vi "LinearFitAnalysis.vi"() -> ()   [LabVIEW 2014]
uses:
  <vilib>/Analysis/NI_AALBase.lvlib
panel:
  out "XY Graph 2":T1(graph)={"X Values"=[-40.353522941082986, -31.05581354762909, -21.758104154175193, -12.460394760721293, -3.162685367267396, 6.135024026186502, 15.4327334196404, 24.730442813094296, 34.02815220654819, 43.32586160000209], "Histogram: h(x)"=[5, 8, 4, 4, 5, 3, 6, 5, 6, 4]}
  out "Histogram":dynamicdata(graph)=[{"t0"=timestamp(-38.357142857142854 s since 1904-01-01), "dt"=13.285714285714286, "Y"=[7.0, 8.0, 5.0, 8.0, 6.0, 8.0, 7.0], "attributes"=variant("NI_ChannelName"=variant(string "Residual (Histogram)"), "NI_ExpIsRelativeTime"=variant(bool TRUE), "NI_ExpStartTimeStamp"=variant(timestamp timestamp(3625242129.7911425 s since 1904-01-01)), "NI_ExpTimeStamp"=variant(timestamp timestamp(3625242129.7911425 s since 1904-01-01)), "NI_ExpXDimension"=variant(string "BIN"), "NI_OriginalChannelName"=variant(string "Residual"))}]
  out "Waveform Graph":dbl[](graph)=[-34.13177225313808, 3.9369650051505545, 2.418342809436112, 33.94654776065637, -28.322445413749968, -23.089453952372995, 46.08339129792877, -35.21104805807906, -14.818260309087094, -11.198957667960379, 38.96344770318322, -27.587731142955796, -18.744026446357005, -7.916162344025565, 41.18155909728465, 1.793736562146897, 37.291403588063744, 35.423104927171835, 0.5951350891973561, 17.922685101270574, -43.76575692098045, -1.442658454638206, 25.124978304862296, 47.97471629672904, 27.058820065498324, -42.86441526358226, 12.858591260563628, 25.163153849942447, -31.604684274195407, -34.659436016289305, 29.822924594912607, -44.9832953564606, 15.032475531004025, -25.15536981059452, 1.165196525852977, -45.002377637809936, -17.765214983464205, -10.510416481626322, 33.44225028666084, 16.6290398135976, -3.536369999863851, -29.84969881839565, 34.743219564744365, 11.20195037721831, -43.93667945124713, -29.06099706997172, 23.60616047154268, 0.7052895578499516, 29.243007457115766, 11.829135227260295]
  out "XY Graph":cluster{i32[], "Array":dbl[]}[](graph)=[{[0, 1, 2, 3, 4, 5, 6, 7, 8, 9, 10, 11, 12, 13, 14, 15, 16, 17, 18, 19, 20, 21, 22, 23, 24, 25, 26, 27, 28, 29, 30, 31, 32, 33, 34, 35, 36, 37, 38, 39, 40, 41, 42, 43, 44, 45, 46, 47, 48, 49], "Array"=[10.092485847483124, 49.451694818548496, 49.22354433561078, 82.04222099960778, 21.063699537978174, 27.58716271213188, 98.05047967521038, 18.046512031979283, 39.72977149374798, 44.63954584765143, 96.09242293157176, 30.83171579820948, 40.96589220758501, 53.08422802269318, 103.47242117678013, 65.37507035441911, 102.16320909311268, 101.58538214499751, 68.04788401979977, 86.66590574464972, 26.26793543517543, 69.88150561429441, 97.73961408657165, 121.87982379121513, 102.25439927276115, 33.621635656457286, 90.63511389337991, 104.23014819553546, 48.752781784174346, 46.98850175485718, 112.76133407883583, 39.24558584023936, 100.5518284404807, 61.654454811658894, 89.26549286088313, 44.38839040999695, 72.91602477711942, 81.46129499173404, 126.70443347279793, 111.18169471251143, 92.30675661182671, 67.28389950607163, 133.1672896019884, 110.91649212723907, 57.06833401155036, 73.23448810560251, 127.19211735989364, 105.58171815897765, 135.4099077710202, 119.28650725394145]}, {[0, 1, 2, 3, 4, 5, 6, 7, 8, 9, 10, 11, 12, 13, 14, 15, 16, 17, 18, 19, 20, 21, 22, 23, 24, 25, 26, 27, 28, 29, 30, 31, 32, 33, 34, 35, 36, 37, 38, 39, 40, 41, 42, 43, 44, 45, 46, 47, 48, 49], "Array"=[44.224258100621206, 45.51472981339794, 46.80520152617467, 48.095673238951406, 49.38614495172814, 50.67661666450488, 51.96708837728161, 53.25756009005834, 54.54803180283508, 55.83850351561181, 57.12897522838854, 58.419446941165276, 59.70991865394201, 61.00039036671875, 62.29086207949548, 63.58133379227221, 64.87180550504894, 66.16227721782568, 67.45274893060241, 68.74322064337915, 70.03369235615588, 71.32416406893262, 72.61463578170935, 73.90510749448609, 75.19557920726282, 76.48605092003955, 77.77652263281628, 79.06699434559302, 80.35746605836975, 81.64793777114649, 82.93840948392322, 84.22888119669996, 85.51935290947668, 86.80982462225342, 88.10029633503015, 89.39076804780689, 90.68123976058362, 91.97171147336036, 93.2621831861371, 94.55265489891383, 95.84312661169056, 97.13359832446729, 98.42407003724402, 99.71454175002076, 101.00501346279749, 102.29548517557423, 103.58595688835096, 104.8764286011277, 106.16690031390442, 107.45737202668116]}]
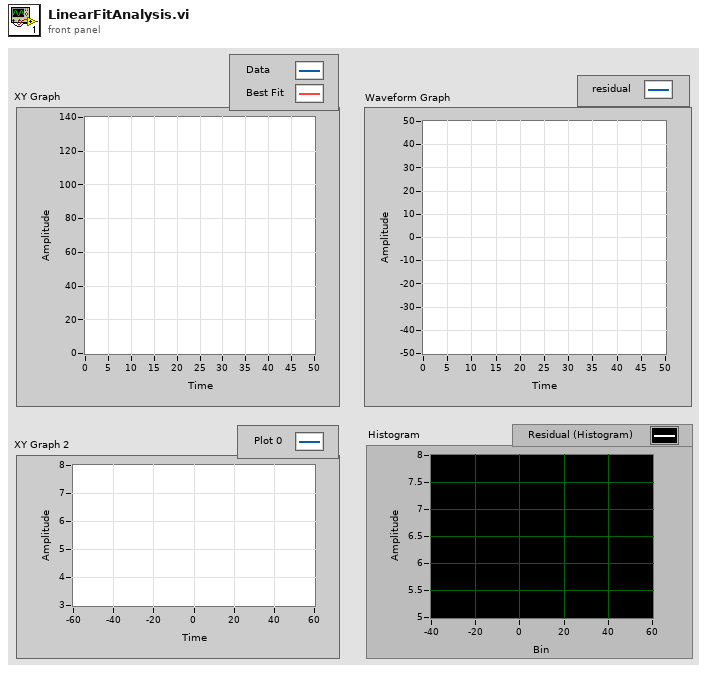
[diagram p1: front panel]
types:
  T1 = cluster{"X Values":dbl[], "Histogram: h(x)":i32[]}
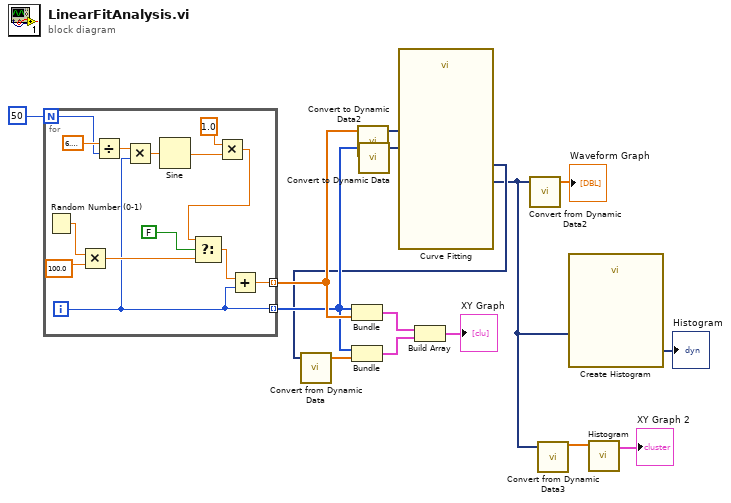
[diagram p0: block diagram]
diagram:
  n1 = for {
    N: 50 -> [w25]
    tunnel: [w20] -> w11 mode=indexing
    tunnel: [w28] -> w13 mode=indexing
    i -> [w20]
    n2 = Random Number (0-1)() -> (number: 0 to 1=w29:dbl)
    n3 = Multiply(x=w29, y=100.0) -> (x*y=w24:dbl)
    n4 = Divide(x=6.283185307179586, y=w25) -> (x/y=w21:dbl)
    n5 = Multiply(x=w21, y=w20) -> (x*y=w19:dbl)
    n6 = Sine(x=w19) -> (sin(x)=w18:dbl)
    n7 = Multiply(x=1.0, y=w18) -> (x*y=w16:dbl)
    n8 = Select(t=w16, s=FALSE, f=w24) -> (s? t:f=w23:dbl)
    n9 = Add(x=w23, y=w20) -> (x+y=w28:dbl)
  }
  n10 = Bundle(w11, w13) -> (w8:cluster{i32[], dbl[]})  [unwired: 1 in]
  n11 = call "Convert to Dynamic Data2"("Array"=w13) -> ("Dynamic Data Type"=w12:dynamicdata)  [unwired: 3 in]
  n12 = call "Convert to Dynamic Data"("Array"=w11) -> ("Dynamic Data Type"=w14:dynamicdata)  [unwired: 3 in]
  n13 = call "Curve Fitting"("Locations"=w14, "Signals"=w12) -> ("residual"=w3:dynamicdata, "best fit"=w10:dynamicdata)  [unwired: 4 in, 4 out]
  n14 = call "Convert from Dynamic Data"("Dynamic Data Type"=w10) -> ("Array"=w9:dbl[])  [unwired: 3 in]
  n15 = Bundle(w11, "Array"=w9) -> (w7:cluster{i32[], "Array":dbl[]})  [unwired: 1 in]
  n16 = Build Array(w8, w7) -> (→"XY Graph":cluster{i32[], "Array":dbl[]}[])
  n17 = call "Convert from Dynamic Data2"("Dynamic Data Type"=w3) -> ("Array"=→"Waveform Graph":dbl[])  [unwired: 3 in]
  n18 = call "Convert from Dynamic Data3"("Dynamic Data Type"=w3) -> ("Array"=w2:dbl[])  [unwired: 3 in]
  n19 = call "Create Histogram"("Signal"=w3) -> ("Histogram"=→"Histogram":dynamicdata)  [unwired: 9 in, 1 out]
  n20 = call <vilib>:"Histogram.vi"("X"=w2) -> ("Histogram Graph"=→"XY Graph 2":T1)  [unwired: 7 in, 3 out]
